vi "PyConv_CreateDiagram.vi"(6 "UID":i32, 7 "PythonConverter_BD in":refnum<class "PyConvBD.lvclass">, 8 "error in":errorcluster, 11 "VI Interpreter in":refnum<class "VI Interpreter.lvclass">) -> (0 "error out":errorcluster, 3 "VI Interpreter out":refnum<class "VI Interpreter.lvclass">, 5 "PythonConverter_BD out":refnum<class "PyConvBD.lvclass">)   [LabVIEW 2014, in "PyConvBD.lvclass"]
uses:
  PyConvBD.lvclass
  VI Interpreter/Classes/VI Interpreter/VI Interpreter.lvclass
  VI Interpreter/Classes/Diagram/Diagram.lvclass
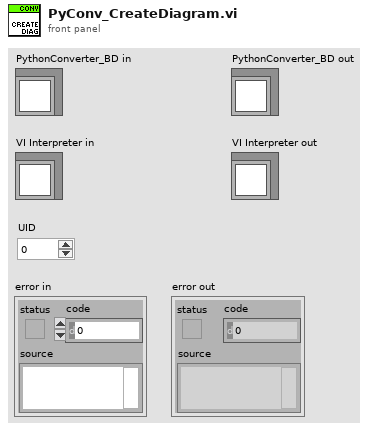
[diagram p1: front panel]
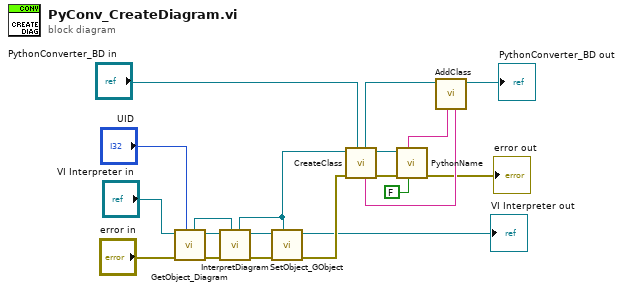
[diagram p0: block diagram]
diagram:
  n1 = call "GetObject_Diagram.vi"("UID"="UID", "error in"="error in", "VI Interpreter in"="VI Interpreter in") -> ("error out"=w9:errorcluster, "VI Interpreter out"=w10:refnum<class "VI Interpreter.lvclass">, "Diagram"=w8:refnum<class "Diagram.lvclass">)  [unwired: 3 in, 1 out]
  n2 = call "InterpretDiagram.vi"("Diagram"=w8, "error in"=w9, "VI Interpreter in"=w10) -> ("error out"=w12:errorcluster, "VI Interpreter out"=w11:refnum<class "VI Interpreter.lvclass">, "Diagram out"=w7:refnum<class "Diagram.lvclass">)  [unwired: 4 in]
  n3 = call "SetObject_GObject.vi"("GObject"=w7, "error in"=w12, "VI Interpreter in"=w11) -> ("error out"=w6:errorcluster, "VI Interpreter out"=→"VI Interpreter out":refnum<class "VI Interpreter.lvclass">)  [unwired: 5 in]
  n4 = call-dynamic "CreateClass.vi"("PythonConverter_BD in"="PythonConverter_BD in", "error in"=w6, "Diagram in"=w7) -> ("error out"=w17:errorcluster, "Diagram out"=w18:refnum<class "Diagram.lvclass">, "diagram"=w13:string, "PythonConverter_BD out"=w19:refnum<class "PyConvBD.lvclass">)  [unwired: 5 in]
  n5 = call-dynamic "PythonName.vi"("add self"=FALSE, "error in"=w17, "Diagram in"=w18) -> ("error out"=→"error out":errorcluster, "UID"=w16:string)  [unwired: 5 in, 2 out]
  n6 = call "AddClass.vi"("definition"=w13, "name"=w16, "PythonConverter_BD in"=w19) -> ("PythonConverter_BD out"=→"PythonConverter_BD out":refnum<class "PyConvBD.lvclass">)  [unwired: 5 in, 1 out]
